vi "Report Cal Measured Power Dll.vi"(0 "CART TCP Connection In":refnum<k5>, 5 "LastFreqCommit":u8, 7 "TxPwrCalChain":u32, 9 "TxPwrCalVal":dbl) -> (4 "CART TCP Connection Out":refnum<k5>, 6 "StatusIsFalse":i16, 8 "DONE?":i16)   [LabVIEW 2011]
uses:
  WLAN/UUT/QCA/NART Constants.vi
panel:
  out "Command Sent":string
  out "TCP Messages":string[](array[string])
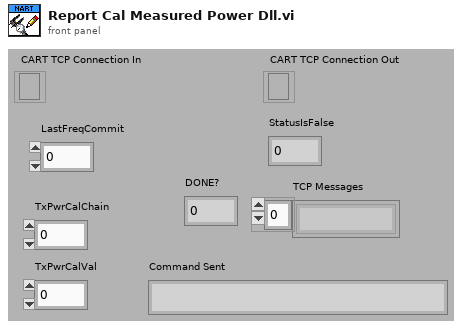
[diagram p1: front panel]
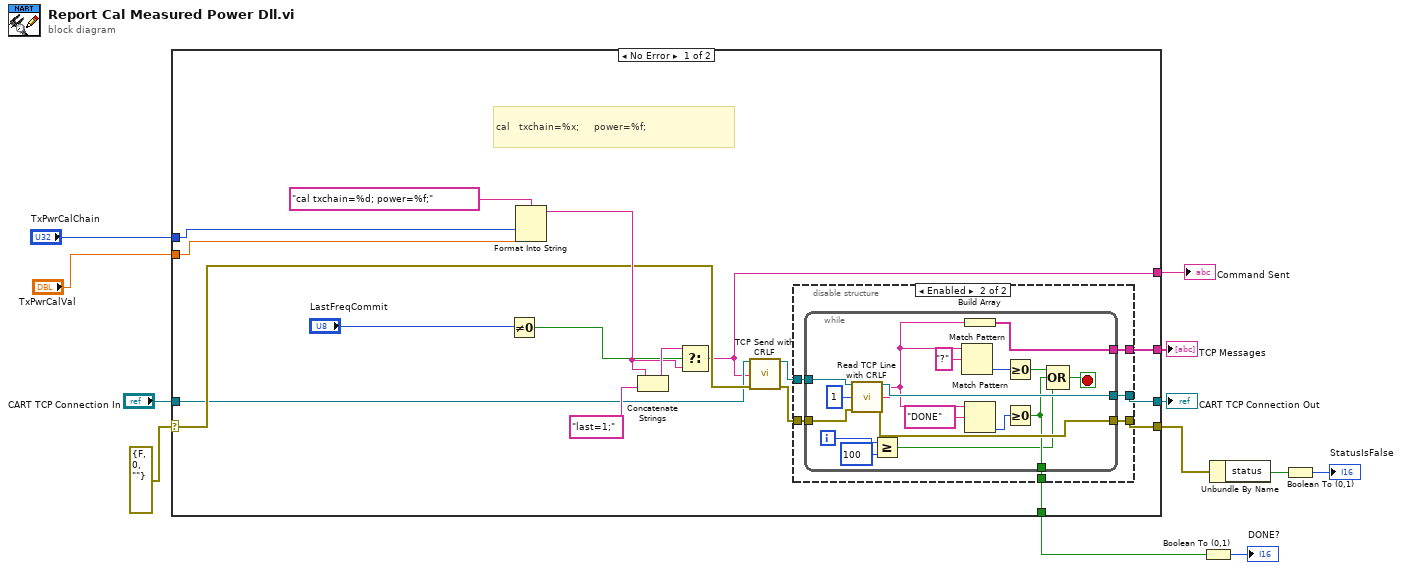
[diagram p0: block diagram]
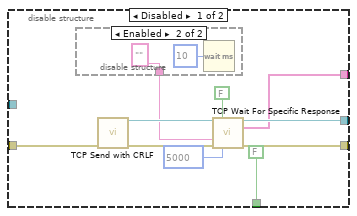
[diagram p2: hidden frame]
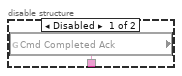
[diagram p3: hidden frame]
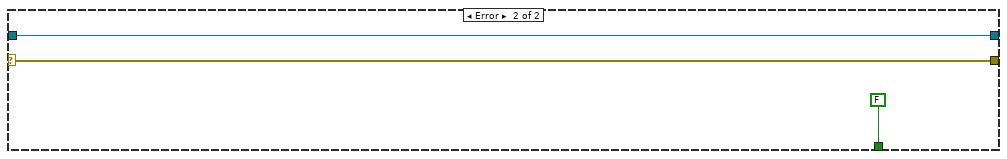
[diagram p4: hidden frame]
diagram:
  n1 = case shown="No Error" errorcluster {"status"=FALSE, "code"=0, "source"=""} ("error in (no error)") {
    selector: errorcluster {"status"=FALSE, "code"=0, "source"=""} ("error in (no error)") -> [w15 w70]
    tunnel: [w28 w70] -> w7
    tunnel: "CART TCP Connection In" -> [w14 w69]
    tunnel: [w29 w69] -> w10
    tunnel: [w27 _] -> w9
    tunnel: [w13 _] -> w8
    tunnel: "TxPwrCalChain" -> [w22 _]
    tunnel: "TxPwrCalVal" -> [w21 _]
    tunnel: [w18 FALSE] -> w1
    frame No Error {
      # "cal   txchain=%x;     power=%f;"
      n2 = Not Equal To 0?(x="LastFreqCommit") -> (x != 0?=w19:bool)
      n3 = Format Into String(format string="cal txchain=%d; power=%f;" ("Name"), w22, w21) -> (resulting string=w23:string)  [unwired: 2 in, 1 out]
      n4 = Concatenate Strings(w23, "last=1;" ("string")) -> (w25:string)
      n5 = Select(t=w25, s=w19, f=w23) -> (s? t:f=w13:string)
      n6 = call "TCP Send with CRLF.vi"("CART TCP Connection"=w14, "data in"=w13, "error IO"=w15) -> ("CART TCP Connection Out"=w17:refnum<k5>, "error out"=w16:errorcluster)  [unwired: 11 in]
      n7 = disable-structure shown="Enabled" {
        disable-tunnel: w16 -> [w40 w50]
        disable-tunnel: [w38 w49] -> w29
        disable-tunnel: [w37 w47] -> w28
        disable-tunnel: [w34 w48] -> w27
        disable-tunnel: [FALSE w46] -> w18
        disable-tunnel: w17 -> [_ w45]
        frame Disabled {
          n8 = disable-structure shown="Enabled" {
            disable-tunnel: [w42 "" ("Expected Message Start (\"\":any)")] -> w32
            frame Disabled {
              n9 = global read "NART Constants.vi" "Cmd Completed Ack"() -> (w42:string)
            }
            frame Enabled {
              n10 = Wait (ms)(milliseconds to wait=u32 10) -> ()  [unwired: 1 out]
            }
          }
          n11 = call "TCP Send with CRLF.vi"("error IO"=w40) -> ("CART TCP Connection"=w41:refnum<k5>, "CART TCP Connection Out"=w39:refnum<k5>, "data in"=w31:string, "error out"=w36:errorcluster)  [unwired: 11 in]
          n12 = call "TCP Wait For Specific Response.vi"("TCP Connection In"=w39, "Next response (t)"=FALSE, "Expected Message Start (\"\":any)"=w32, "error in"=w36, "Timeout (250 ms)"=5000) -> ("TCP Connection Out"=w38:refnum<k5>, "TCP Messages"=w34:string[], "error out"=w37:errorcluster)  [unwired: 7 in, 1 out]
        }
        frame Enabled {
          n13 = while {
            tunnel: w50 -> [w66]
            tunnel: w45 -> [w65]
            tunnel: [w64] -> w49
            tunnel: [w63] -> w48
            tunnel: [w62] -> w47
            tunnel: [w53] -> w46
            i -> [w56]
            stop <- w51 stop-if-true
            n14 = call "Read TCP Line with CRLF.vi"("TCP Connection In"=w65, "timeout ms (100)"=1, "error in"=w66) -> ("TCP Connection Out"=w64:refnum<k5>, "TCP Line"=w59:string, "error out"=w62:errorcluster)  [unwired: 10 in]
            n15 = Greater Or Equal?(x=w56, y=100) -> (x >= y?=w52:bool)
            n16 = Match Pattern(string=w59, regular expression="?") -> (offset past match=w60:i32)  [unwired: 1 in, 3 out]
            n17 = Build Array(w59) -> (w63:string[])
            n18 = Match Pattern(string=w59, regular expression="DONE") -> (offset past match=w57:i32)  [unwired: 1 in, 3 out]
            n19 = Greater Or Equal To 0?(x=w60) -> (x >= 0?=w54:bool)
            n20 = Greater Or Equal To 0?(x=w57) -> (x >= 0?=w53:bool)
            n21 = Compound Arithmetic op=OR(w54, w53, w52) -> (w51:bool)
          }
        }
      }
    }
    frame Error {
    }
  }
  "CART TCP Connection Out" <- w10
  "TCP Messages" <- w9
  "Command Sent" <- w8
  n22 = Boolean To (0,1)(Boolean=w1) -> (0, 1=→"DONE?":i16)
  n23 = Unbundle By Name(w7) -> ("status"=w5:bool)
  n24 = Boolean To (0,1)(Boolean=w5) -> (0, 1=→"StatusIsFalse":i16)
